vi "参数配置表.vi"() -> ()   [LabVIEW 2016, in "数据传输系统-05.lvlib"]
uses:
  <vilib>/Utility/miscctls.llb/LVPointTypeDef.ctl
  <vilib>/ptbypt/NI_PtbyPt.lvlib
panel:
  in  "加密传输":bool
  in  "数据库类型":enum16{"Access", "SQLite"}(ring)
  in  "应用环境":enum16{"STD", "GB212"}(ring)
  in  "屏蔽维护数据":bool
  in  "数据发送延时时间/s":i32
  in  "判断数据反馈":enum16{"非严格判断", "严格判断", "不判断"}(ring)
  in  "仪器参数发送":bool
  in  "地表水/污染源":bool
  in  "间隔时间/分钟":i32
  in  "数据发送通道":enum16{"TCP", "VISA"}(ring)
  in  "数据发送协议":enum16{"2005-212协议", "2017-212协议"}(ring)=enum."2017-212协议"
  in  "数据触发上传方式":enum16{"出数即刻发送", "间隔时间发送", "整点发送"}(ring)
  in  "数据组合发送":bool
  in  "日志、参数发送":bool
  in  "2011发送":bool
  in  "返回":bool
  out "配置表格":string[][](table)
  in  "参数数值":T1={"CODMn"=TRUE, "CODCr"=TRUE, "DO"=TRUE, "铜"=TRUE, "PH"=TRUE, "氨氮"=TRUE, "比电导率"=TRUE, "水温"=TRUE, "COD"=TRUE, "浊度"=TRUE, "总氮"=TRUE, "总磷"=TRUE, "叶绿素a"=TRUE, "藻密度"=TRUE, "水位"=TRUE, "流速"=TRUE, "瞬时流量"=TRUE, "累积流量"=TRUE, "亚硝氮"=TRUE, "硫化物"=TRUE, "ORP"=TRUE, "铅"=TRUE, "镉"=TRUE, "锌"=TRUE, "镍"=TRUE, "锰"=TRUE, "汞"=TRUE, "气温"=TRUE, "气压"=TRUE, "风速"=TRUE, "风向"=TRUE, "盐度"=TRUE, "磷酸盐"=TRUE, "硝氮"=TRUE, "氟化物"=TRUE}
  # "因子编码，单位配置，上传功能码，小时、质控数据上传触发方式"
  # "参数配置"
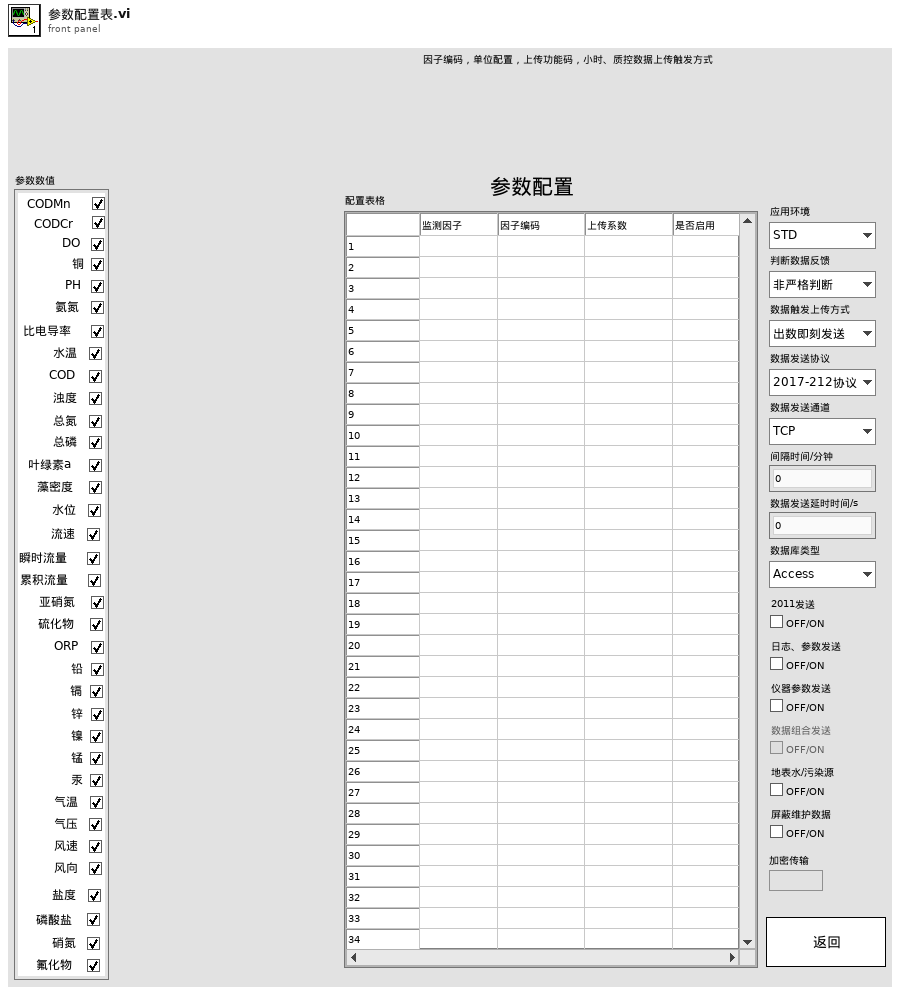
[diagram p1: front panel]
types:
  T1 = cluster{"CODMn":bool, "CODCr":bool, "DO":bool, "铜":bool, "PH":bool, "氨氮":bool, "比电导率":bool, "水温":bool, "COD":bool, "浊度":bool, "总氮":bool, "总磷":bool, "叶绿素a":bool, "藻密度":bool, "水位":bool, "流速":bool, "瞬时流量":bool, "累积流量":bool, "亚硝氮":bool, "硫化物":bool, "ORP":bool, "铅":bool, "镉":bool, "锌":bool, "镍":bool, "锰":bool, "汞":bool, "气温":bool, "气压":bool, "风速":bool, "风向":bool, "盐度":bool, "磷酸盐":bool, "硝氮":bool, "氟化物":bool}
  T2 = typedef "LVPointTypeDef.ctl" = cluster{"Horizontal":i16, "Vertical":i16}
  T3 = cluster{"[0]":string, "[1]":string, "[2]":string, "[3]":string, "[4]":string, "[5]":string, "[6]":string, "[7]":string, "[8]":string, "[9]":string, "[10]":string, "[11]":string, "[12]":string, "[13]":string, "[14]":string, "[15]":string, "[16]":string, "[17]":string, "[18]":string, "[19]":string, "[20]":string, "[21]":string, "[22]":string, "[23]":string, "[24]":string, "[25]":string, "[26]":string, "[27]":string, "[28]":string, "[29]":string, "[30]":string, "[31]":string, "[32]":string, "[33]":string, "[34]":string}
  T4 = enum8{"Enabled", "Disabled", "Disabled and Grayed Out"}
  T5 = typedef "LVRowAndColumnTypeDef.ctl" = cluster{"Row":i32, "Column":i32}
  T6 = cluster{"[0]":string, "[1]":string, "[2]":string, "[3]":string, "[4]":string, "[5]":string, "[6]":string}
  T7 = cluster{"[0]":string, "[1]":string, "[2]":string, "[3]":string, "[4]":string, "[5]":string, "[6]":string, "[7]":string, "[8]":string, "[9]":string, "[10]":string, "[11]":string, "[12]":string}
  T8 = cluster{"[0]":string, "[1]":string, "[2]":string, "[3]":string, "[4]":string, "[5]":string, "[6]":string, "[7]":string, "[8]":string, "[9]":string, "[10]":string, "[11]":string, "[12]":string, "[13]":string}
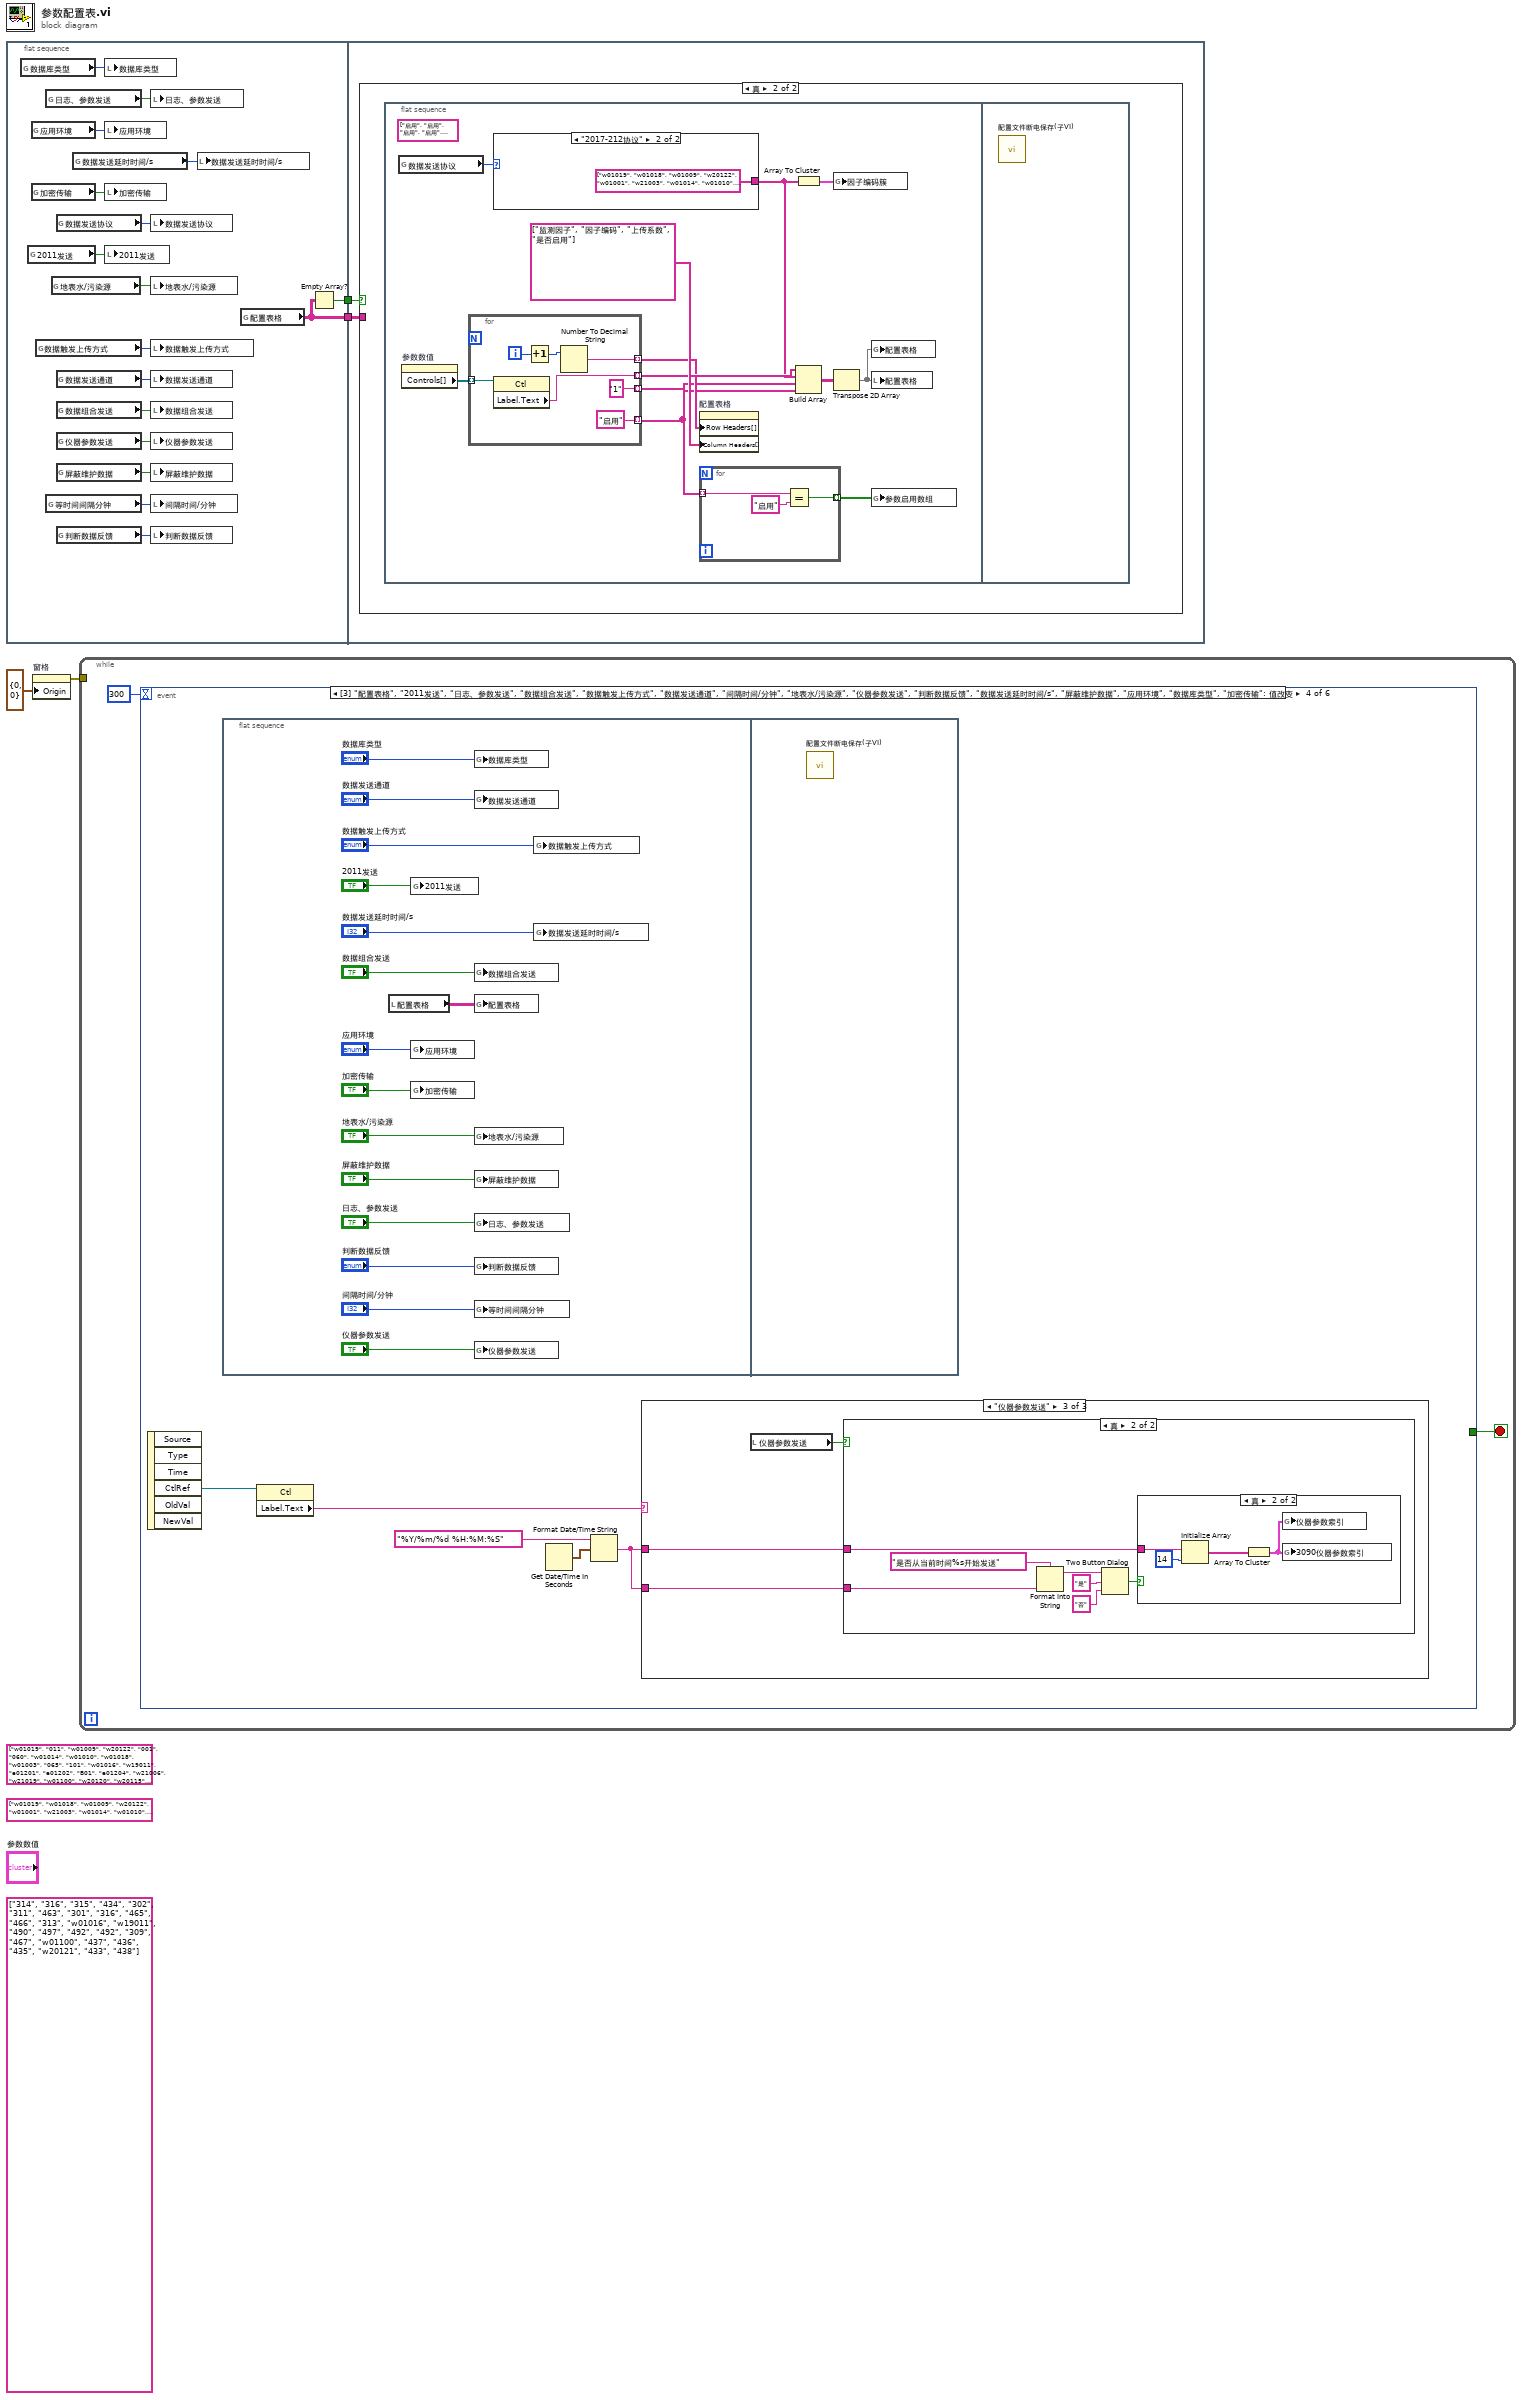
[diagram p0: block diagram]
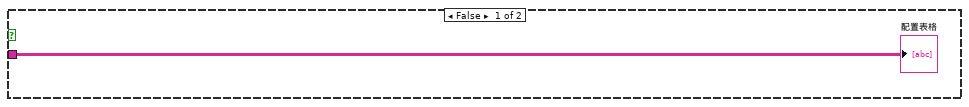
[diagram p2: hidden frame]
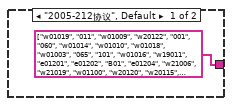
[diagram p3: hidden frame]
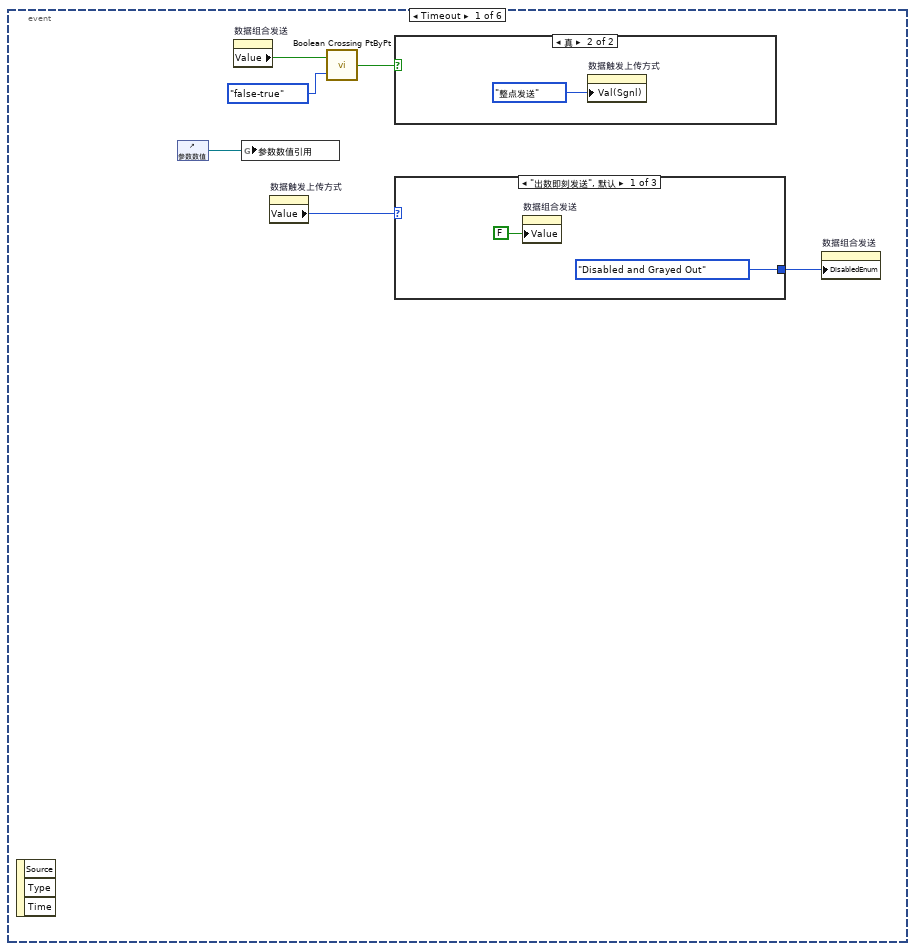
[diagram p4: hidden frame]
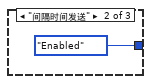
[diagram p6: hidden frame]
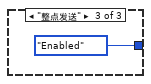
[diagram p7: hidden frame]
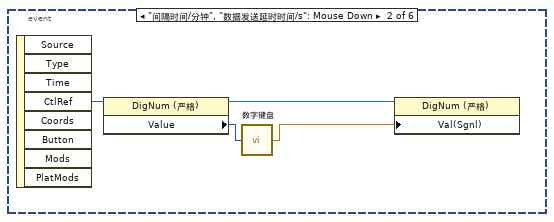
[diagram p8: hidden frame]
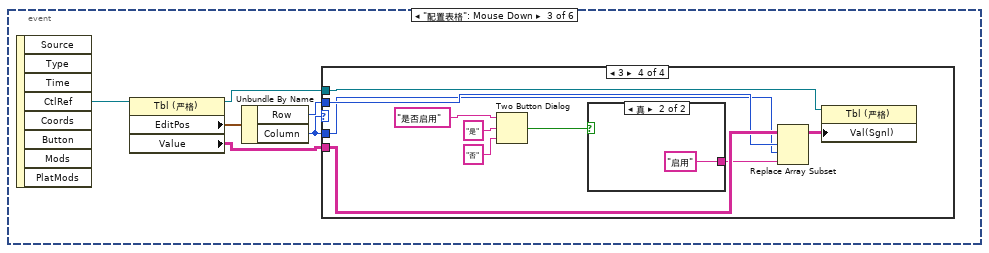
[diagram p9: hidden frame]
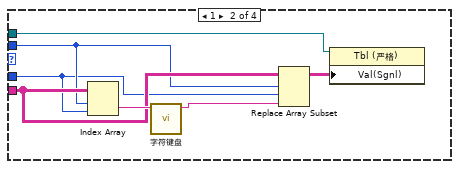
[diagram p11: hidden frame]
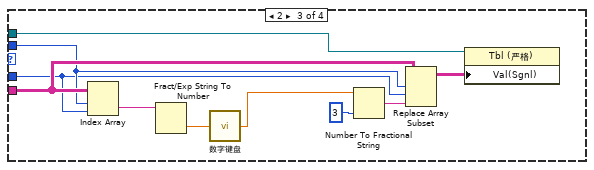
[diagram p12: hidden frame]
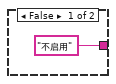
[diagram p13: hidden frame]
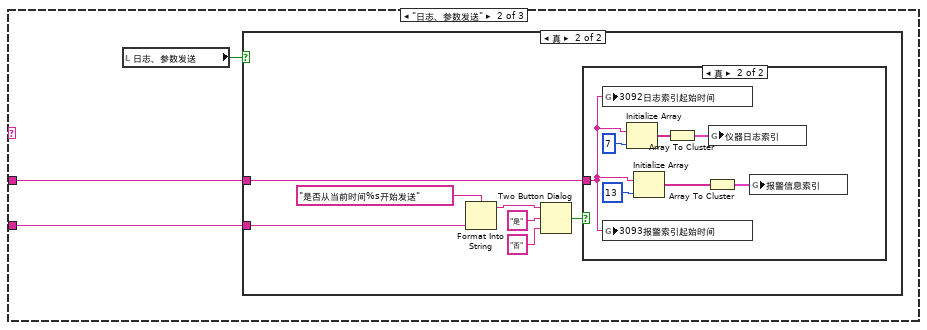
[diagram p15: hidden frame]
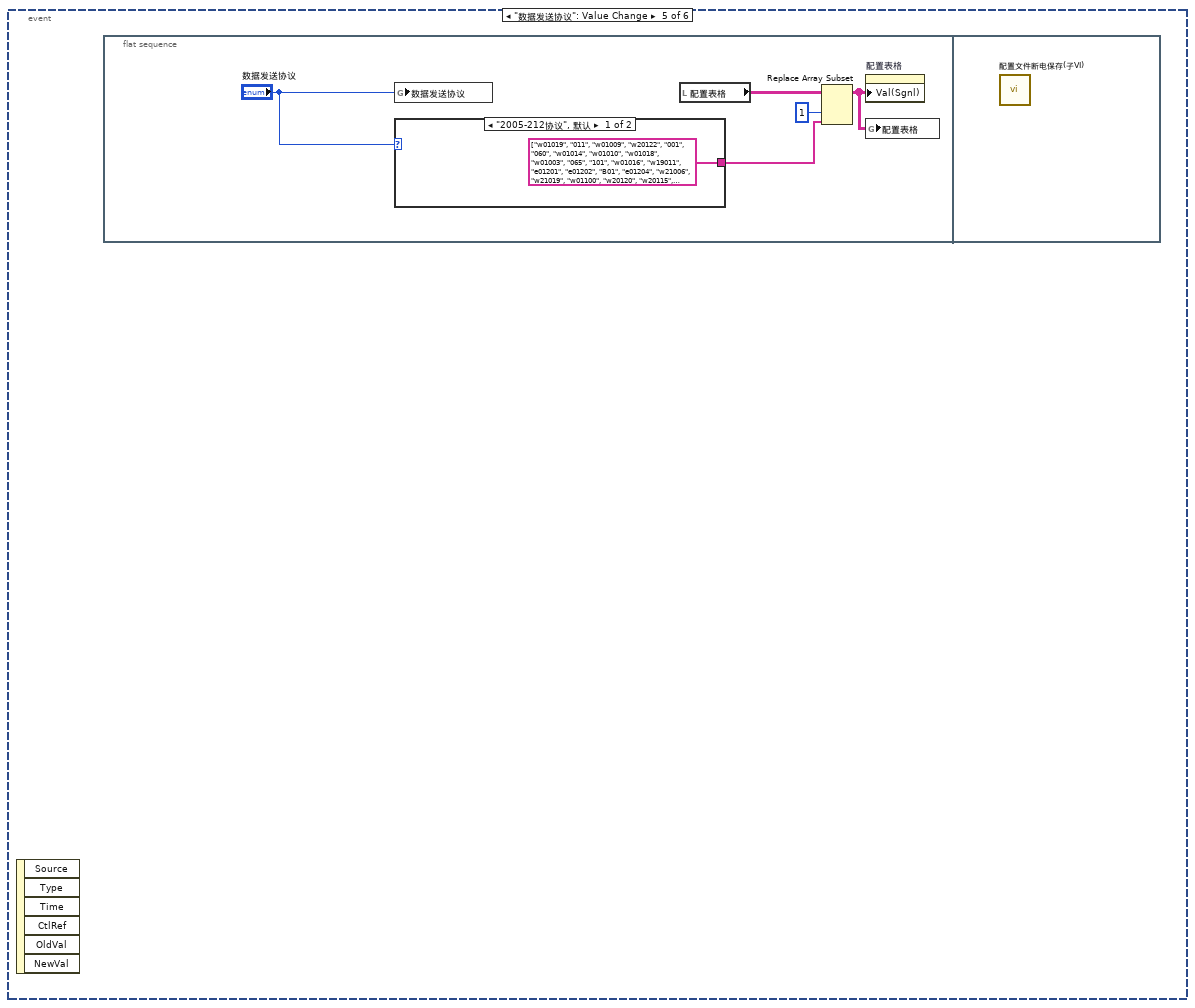
[diagram p20: hidden frame]
diagram:
  (unwired) string[] ["w01019", "011", "w01009", "w20122", "001", "060", "w01014", "w01010", "w01018", "w01003", "065", "101", "w01016", "w19011", "e01201", "e01202", "B01", "e01204", "w21006", "w21019", "w01100", "w20120", "w20115", "w20123", "w20121", "w20124", "w20111", "a01001", "a01006", "a01007", "a01008", "w01002", "w21015", "w21007", "w21017"]
  (unwired) string[] ["w01019", "w01018", "w01009", "w20122", "w01001", "w21003", "w01014", "w01010", "w01018", "w01003", "w21001", "w21011", "w01016", "w19011", "e01201", "e01202", "e01203", "e01204", "w21006", "w21019", "w01100", "w20120", "w20115", "w20123", "w20121", "w20124", "w20111", "a01001", "a01006", "a01007", "a01008", "w01002", "w21015", "w21007", "w21017"]
  (unwired) string[] ["314", "316", "315", "434", "302", "311", "463", "301", "316", "465", "466", "313", "w01016", "w19011", "490", "497", "492", "492", "309", "467", "w01100", "437", "436", "435", "w20121", "433", "438"]
  n1 = flat-sequence {
    tunnel: [w14] -> w2
    tunnel: [w13] -> w1
    tunnel: w2 -> [w23]
    tunnel: w1 -> [w22]
    frame #0 {
      n2 = global read "断电保存全局.vi" "数据库类型"() -> (w6:enum16{"Access", "SQLite"})
      n3 = global read "断电保存全局.vi" "2011发送"() -> (w21:bool)
      n4 = global read "断电保存全局.vi" "应用环境"() -> (w7:enum16{"STD", "GB212"})
      n5 = global read "断电保存全局.vi" "加密传输"() -> (w5:bool)
      n6 = global read "断电保存全局.vi" "数据触发上传方式"() -> (w17:enum16{"出数即刻发送", "间隔时间发送", "整点发送"})
      n7 = global read "断电保存全局.vi" "日志、参数发送"() -> (w19:bool)
      n8 = global read "断电保存全局.vi" "等时间间隔分钟"() -> (w12:i32)
      n9 = global read "断电保存全局.vi" "地表水/污染源"() -> (w11:bool)
      n10 = global read "断电保存全局.vi" "数据发送协议"() -> (w15:enum16{"2005-212协议", "2017-212协议"})
      n11 = global read "断电保存全局.vi" "数据发送通道"() -> (w16:enum16{"TCP", "VISA"})
      n12 = global read "断电保存全局.vi" "数据组合发送"() -> (w18:bool)
      n13 = global read "断电保存全局.vi" "仪器参数发送"() -> (w10:bool)
      n14 = global read "断电保存全局.vi" "屏蔽维护数据"() -> (w8:bool)
      n15 = global read "断电保存全局.vi" "判断数据反馈"() -> (w20:enum16{"非严格判断", "严格判断", "不判断"})
      n16 = global read "断电保存全局.vi" "数据发送延时时间/s"() -> (w9:i32)
      n17 = local write "数据库类型"(w6) -> ()
      n18 = local write "应用环境"(w7) -> ()
      n19 = local write "加密传输"(w5) -> ()
      n20 = local write "2011发送"(w21) -> ()
      n21 = local write "日志、参数发送"(w19) -> ()
      n22 = local write "数据发送协议"(w15) -> ()
      n23 = local write "地表水/污染源"(w11) -> ()
      n24 = local write "数据触发上传方式"(w17) -> ()
      n25 = local write "数据发送通道"(w16) -> ()
      n26 = local write "数据组合发送"(w18) -> ()
      n27 = local write "仪器参数发送"(w10) -> ()
      n28 = local write "屏蔽维护数据"(w8) -> ()
      n29 = local write "间隔时间/分钟"(w12) -> ()
      n30 = local write "判断数据反馈"(w20) -> ()
      n31 = local write "数据发送延时时间/s"(w9) -> ()
      n32 = global read "断电保存全局.vi" "配置表格"() -> (w13:string[][])
      n33 = Empty Array?(array=w13) -> (empty?=w14:bool)
    }
    frame #1 {
      n34 = case shown="真" w23 {
        tunnel: w22 -> [w24 _]
        frame False {
          "配置表格" <- w24
        }
        frame True {
          n35 = flat-sequence {
            frame #0 {
              (unwired) string[] ["启用", "启用", "启用", "启用", "启用", "启用", "启用", "启用", "启用", "启用", "启用", "启用", "启用", "启用", "启用", "启用", "启用", "启用", "启用", "启用", "启用", "启用", "启用", "启用", "启用", "启用", "启用"]
              n36 = global read "断电保存全局.vi" "数据发送协议"() -> (w30:enum16{"2005-212协议", "2017-212协议"})
              n37 = property on="参数数值" class="Clust (严格)"() -> ("Controls[]"=w32:refnum<vi>[])  [unwired: 2 in, 2 out]
              n38 = for {
                tunnel: w32 -> [w48] mode=indexing
                tunnel: [w47] -> w34 mode=indexing
                tunnel: [w45] -> w33 mode=indexing
                tunnel: ["1"] -> w27 mode=indexing
                tunnel: ["启用"] -> w25 mode=indexing
                i -> [w46]
                n39 = property class="Ctl"(reference=w48) -> ("Label.Text"=w47:string)  [unwired: 1 in, 2 out]
                n40 = Increment(x=w46) -> (x+1=w44:i32)
                n41 = Number To Decimal String(number=w44) -> (decimal integer string=w45:string)  [unwired: 1 in]
              }
              n42 = case shown="\"2017-212协议\"" w30 {
                tunnel: [string[] ["w01019", "011", "w01009", "w20122", "001", "060", "w01014", "w01010", "w01018", "w01003", "065", "101", "w01016", "w19011", "e01201", "e01202", "B01", "e01204", "w21006", "w21019", "w01100", "w20120", "w20115", "w20123", "w20121", "w20124", "w20111", "a01001", "a01006", "a01007", "a01008", "w01002", "w21015", "w21007", "w21017"] string[] ["w01019", "w01018", "w01009", "w20122", "w01001", "w21003", "w01014", "w01010", "w01018", "w01003", "w21001", "w21011", "w01016", "w19011", "e01201", "e01202", "e01203", "e01204", "w21006", "w21019", "w01100", "w20120", "w20115", "w20123", "w20121", "w20124", "w20111", "a01001", "a01006", "a01007", "a01008", "w01002", "w21015", "w21007", "w21017"]] -> w28
                frame "2005-212协议", Default {
                }
                frame "2017-212协议" {
                }
              }
              n43 = property on="配置表格" class="Tbl (严格)"("Row Headers[]"=w33, "Column Headers[]"=string[] ["监测因子", "因子编码", "上传系数", "是否启用"]) -> ()  [unwired: 2 in, 2 out]
              n44 = for {
                tunnel: w25 -> [w39] mode=indexing
                tunnel: [w37] -> w26 mode=indexing
                n45 = Equal?(x=w39, y="启用") -> (x = y?=w37:bool)
              }
              n46 = Array To Cluster(array=w28) -> (cluster=w29:T3)
              n47 = Build Array(w34, w28, w27, w25) -> (w36:string[][])
              n48 = global write "断电保存全局.vi" "因子编码簇"(w29) -> ()
              n49 = Transpose 2D Array(2D array=w36) -> (transposed array=w31:string[][])
              n50 = global write "断电保存全局.vi" "配置表格"(w31) -> ()
              n51 = local write "配置表格"(w31) -> ()
              n52 = global write "断电保存全局.vi" "参数启用数组"(w26) -> ()
            }
            frame #1 {
              n53 = call "配置文件断电保存(子VI).vi"() -> ()  [unwired: 12 in]
            }
          }
        }
      }
    }
  }
  n54 = property on="窗格" class="Pane"("Origin"=T2 {"Horizontal"=0, "Vertical"=0} ("原点")) -> (error out=w4:errorcluster)  [unwired: 2 in, 1 out]
  n55 = while {
    tunnel: w4 -> [_]
    stop <- w49 stop-if-true
    n56 = event shown="[3] \"配置表格\", \"2011发送\", \"日志、参数发送\", \"数据组合发送\", \"数据触发上传方式\", \"数据发送通道\", \"间隔时间/分钟\", \"地表水/污染源\", \"仪器参数发送\", \"判断数据反馈\", \"数据发送延时时间/s\", \"屏蔽维护数据\", \"应用环境\", \"数据库类型\", \"加密传输\": 值改变" {
      selector: _ -> [_ _ _ _ _ _]
      dyn-events: _ -> [_ _ _ _ _ _]
      timeout: 300 -> [_ _ _ _ _ _]
      tunnel: [_ _ _ _ _ TRUE] -> w49
      event Timeout {
        n57 = event-data() -> ()  [unwired: 1 in, 3 out]
        n58 = control-ref of="参数数值"() -> (w51:refnum<vi>)
        n59 = property on="数据组合发送" class="Bool (严格)"() -> ("Value"=w54:bool)  [unwired: 2 in, 2 out]
        n60 = global write "断电保存全局.vi" "参数数值引用"(w51) -> ()
        n61 = property on="数据触发上传方式" class="Enum (严格)"() -> ("Value"=w56:enum16{"出数即刻发送", "间隔时间发送", "整点发送"})  [unwired: 2 in, 2 out]
        n62 = call <vilib>:"Boolean Crossing PtByPt.vi"("direction"=enum16{"either", "false-true", "true-false"}."false-true", "input"=w54) -> ("crossing"=w52:bool)  [unwired: 1 in]
        n63 = case shown="真" w52 {
          frame False {
          }
          frame True {
            n64 = property on="数据触发上传方式" class="Enum (严格)"("Val(Sgnl)"=enum16{"出数即刻发送", "间隔时间发送", "整点发送"}."整点发送" ("值(信号)")) -> ()  [unwired: 2 in, 2 out]
          }
        }
        n65 = case shown="\"出数即刻发送\", 默认" w56 {
          tunnel: [T4."Disabled and Grayed Out" ("禁用") T4."Enabled" ("禁用") T4."Enabled" ("禁用")] -> w55
          frame "出数即刻发送", Default {
            n66 = property on="数据组合发送" class="Bool (严格)"("Value"=FALSE ("值(信号)")) -> ()  [unwired: 2 in, 2 out]
          }
          frame "间隔时间发送" {
          }
          frame "整点发送" {
          }
        }
        n67 = property on="数据组合发送" class="Bool (严格)"("DisabledEnum"=w55) -> ()  [unwired: 2 in, 2 out]
      }
      event "间隔时间/分钟", "数据发送延时时间/s": Mouse Down {
        n68 = event-data() -> ("CtlRef"=w65:refnum<vi>)  [unwired: 1 in, 7 out]
        n69 = property class="DigNum (严格)"(reference=w65) -> (reference out=w63:refnum<vi>, "Value"=w64:i32)  [unwired: 1 in, 1 out]
        n70 = call "数字键盘.vi"("OldNumber"=w64) -> ("NewNumber"=w62:sgl)
        n71 = property class="DigNum (严格)"(reference=w63, "Val(Sgnl)"=w62) -> ()  [unwired: 1 in, 2 out]
      }
      event "配置表格": Mouse Down {
        n72 = event-data() -> ("CtlRef"=w71:refnum<vi>)  [unwired: 1 in, 7 out]
        n73 = property class="Tbl (严格)"(reference=w71) -> (reference out=w67:refnum<vi>, "EditPos"=w70:T5, "Value"=w69:string[][])  [unwired: 1 in, 1 out]
        n74 = Unbundle By Name(w70) -> ("Row"=w68:i32, "Column"=w66:i32)
        n75 = case shown="3" w66 {
          tunnel: w69 -> [_ w77 w88 w92]
          tunnel: w68 -> [_ w76 w87 w91]
          tunnel: w66 -> [_ w75 w86 w90]
          tunnel: w67 -> [_ w73 w85 w93]
          frame 0, Default {
          }
          frame 1 {
            n76 = Index Array(array=w77, index (row)=w76, index (col)=w75) -> (element=w78:string)
            n77 = call "字符键盘.vi"("原值"=w78) -> ("x+y"=w74:string)  [unwired: 10 in]
            n78 = Replace Array Subset(array=w77, new element=w74, index (row)=w76, index (col)=w75) -> (w72:string[][])
            n79 = property class="Tbl (严格)"(reference=w73, "Val(Sgnl)"=w72) -> ()  [unwired: 1 in, 2 out]
          }
          frame 2 {
            n80 = Index Array(array=w88, index (row)=w87, index (col)=w86) -> (element=w83:string)
            n81 = Fract/Exp String To Number(string=w83) -> (number=w82:dbl)  [unwired: 3 in, 1 out]
            n82 = call "数字键盘.vi"("OldNumber"=w82) -> ("NewNumber"=w81:sgl)
            n83 = Number To Fractional String(number=w81, precision (6)=i16 3 ("精度(6)")) -> (F-format string=w80:string)  [unwired: 2 in]
            n84 = Replace Array Subset(array=w88, new element=w80, index (row)=w87, index (col)=w86) -> (w84:string[][])
            n85 = property class="Tbl (严格)"(reference=w85, "Val(Sgnl)"=w84) -> ()  [unwired: 1 in, 2 out]
          }
          frame 3 {
            n86 = Two Button Dialog(message="是否启用" ("消息"), 1:"否" ("F按钮名称（“取消”）"), 2:"是" ("T按钮名称（“确定”）")) -> (T button?=w95:bool)
            n87 = case shown="真" w95 {
              tunnel: ["不启用" "启用"] -> w89
              frame False {
              }
              frame True {
              }
            }
            n88 = Replace Array Subset(array=w92, new element=w89, index (row)=w91, index (col)=w90) -> (w94:string[][])
            n89 = property class="Tbl (严格)"(reference=w93, "Val(Sgnl)"=w94) -> ()  [unwired: 1 in, 2 out]
          }
        }
      }
      event "配置表格", "2011发送", "日志、参数发送", "数据组合发送", "数据触发上传方式", "数据发送通道", "间隔时间/分钟", "地表水/污染源", "仪器参数发送", "判断数据反馈", "数据发送延时时间/s", "屏蔽维护数据", "应用环境", "数据库类型", "加密传输": Value Change {
        n90 = event-data() -> ("CtlRef"=w105:refnum<vi>)  [unwired: 1 in, 5 out]
        n91 = flat-sequence {
          frame #0 {
            n92 = local read "配置表格"() -> (w151:string[][])
            n93 = global write "断电保存全局.vi" "2011发送"("2011发送") -> ()
            n94 = global write "断电保存全局.vi" "应用环境"("应用环境") -> ()
            n95 = global write "断电保存全局.vi" "加密传输"("加密传输") -> ()
            n96 = global write "断电保存全局.vi" "数据库类型"("数据库类型") -> ()
            n97 = global write "断电保存全局.vi" "数据发送通道"("数据发送通道") -> ()
            n98 = global write "断电保存全局.vi" "数据组合发送"("数据组合发送") -> ()
            n99 = global write "断电保存全局.vi" "配置表格"(w151) -> ()
            n100 = global write "断电保存全局.vi" "地表水/污染源"("地表水/污染源") -> ()
            n101 = global write "断电保存全局.vi" "屏蔽维护数据"("屏蔽维护数据") -> ()
            n102 = global write "断电保存全局.vi" "日志、参数发送"("日志、参数发送") -> ()
            n103 = global write "断电保存全局.vi" "判断数据反馈"("判断数据反馈") -> ()
            n104 = global write "断电保存全局.vi" "等时间间隔分钟"("间隔时间/分钟") -> ()
            n105 = global write "断电保存全局.vi" "仪器参数发送"("仪器参数发送") -> ()
            n106 = global write "断电保存全局.vi" "数据触发上传方式"("数据触发上传方式") -> ()
            n107 = global write "断电保存全局.vi" "数据发送延时时间/s"("数据发送延时时间/s") -> ()
          }
          frame #1 {
            n108 = call "配置文件断电保存(子VI).vi"() -> ()  [unwired: 12 in]
          }
        }
        n109 = property class="Ctl"(reference=w105) -> ("Label.Text"=w104:string)  [unwired: 1 in, 2 out]
        n110 = Get Date/Time In Seconds() -> (seconds since 1Jan1904=w103:timestamp)
        n111 = Format Date/Time String(time format string (%c)="%Y/%m/%d %H:%M:%S" ("时间格式字符串(%c)"), seconds (now)=w103) -> (date/time string=w101:string)  [unwired: 1 in]
        n112 = case shown="\"仪器参数发送\"" w104 {
          tunnel: w101 -> [_ w107 w124]
          tunnel: w101 -> [_ w106 w123]
          frame "假", Default {
          }
          frame "日志、参数发送" {
            n113 = local read "日志、参数发送"() -> (w108:bool)
            n114 = case shown="真" w108 {
              tunnel: w107 -> [_ w112]
              tunnel: w106 -> [_ w110]
              frame False {
              }
              frame True {
                n115 = Format Into String(format string="是否从当前时间%s开始发送" ("消息"), w110) -> (resulting string=w109:string)  [unwired: 2 in, 1 out]
                n116 = Two Button Dialog(message=w109, 1:"否" ("F按钮名称（“取消”）"), 2:"是" ("T按钮名称（“确定”）")) -> (T button?=w113:bool)
                n117 = case shown="真" w113 {
                  tunnel: w112 -> [_ w116]
                  frame False {
                  }
                  frame True {
                    n118 = global write "全局 时间2.vi" "3092日志索引起始时间"(w116) -> ()
                    n119 = global write "全局 时间2.vi" "3093报警索引起始时间"(w116) -> ()
                    n120 = Initialize Array(w116, 7 ("维数大小")) -> (w117:string[])
                    n121 = Initialize Array(w116, 13 ("维数大小")) -> (w120:string[])
                    n122 = Array To Cluster(array=w117) -> (cluster=w118:T6)
                    n123 = Array To Cluster(array=w120) -> (cluster=w119:T7)
                    n124 = global write "全局 时间2.vi" "仪器日志索引"(w118) -> ()
                    n125 = global write "全局 时间2.vi" "报警信息索引"(w119) -> ()
                  }
                }
              }
            }
          }
          frame "仪器参数发送" {
            n126 = local read "仪器参数发送"() -> (w125:bool)
            n127 = case shown="真" w125 {
              tunnel: w124 -> [_ w129]
              tunnel: w123 -> [_ w127]
              frame False {
              }
              frame True {
                n128 = Format Into String(format string="是否从当前时间%s开始发送" ("消息"), w127) -> (resulting string=w126:string)  [unwired: 2 in, 1 out]
                n129 = Two Button Dialog(message=w126, 1:"否" ("F按钮名称（“取消”）"), 2:"是" ("T按钮名称（“确定”）")) -> (T button?=w130:bool)
                n130 = case shown="真" w130 {
                  tunnel: w129 -> [_ w134]
                  frame False {
                  }
                  frame True {
                    n131 = Initialize Array(w134, 14 ("维数大小")) -> (w136:string[])
                    n132 = Array To Cluster(array=w136) -> (cluster=w133:T8)
                    n133 = global write "全局 时间2.vi" "仪器参数索引"(w133) -> ()
                    n134 = global write "全局 时间2.vi" "3090仪器参数索引"(w133) -> ()
                  }
                }
              }
            }
          }
        }
      }
      event "数据发送协议": Value Change {
        n135 = event-data() -> ()  [unwired: 1 in, 6 out]
        n136 = flat-sequence {
          frame #0 {
            n137 = global write "断电保存全局.vi" "数据发送协议"("数据发送协议") -> ()
            n138 = case shown="\"2005-212协议\", 默认" "数据发送协议" {
              tunnel: [string[] ["w01019", "011", "w01009", "w20122", "001", "060", "w01014", "w01010", "w01018", "w01003", "065", "101", "w01016", "w19011", "e01201", "e01202", "B01", "e01204", "w21006", "w21019", "w01100", "w20120", "w20115", "w20123", "w20121", "w20124", "w20111", "a01001", "a01006", "a01007", "a01008", "w01002", "w21015", "w21007", "w21017"] string[] ["w01019", "w01018", "w01009", "w20122", "w01001", "w21003", "w01014", "w01010", "w01018", "w01003", "w21001", "w21011", "w01016", "w19011", "e01201", "e01202", "e01203", "e01204", "w21006", "w21019", "w01100", "w20120", "w20115", "w20123", "w20121", "w20124", "w20111", "a01001", "a01006", "a01007", "a01008", "w01002", "w21015", "w21007", "w21017"]] -> w154
              frame "2005-212协议", Default {
              }
              frame "2017-212协议" {
              }
            }
            n139 = local read "配置表格"() -> (w155:string[][])
            n140 = Replace Array Subset(array=w155, new element=w154, index (col)=1 ("禁用的索引 (列)")) -> (w152:string[][])  [unwired: 1 in]
            n141 = property on="配置表格" class="Tbl (严格)"("Val(Sgnl)"=w152) -> ()  [unwired: 2 in, 2 out]
            n142 = global write "断电保存全局.vi" "配置表格"(w152) -> ()
          }
          frame #1 {
            n143 = call "配置文件断电保存(子VI).vi"() -> ()  [unwired: 12 in]
          }
        }
      }
      event "返回": Value Change; Panel Close {
        n144 = event-data() -> ()  [unwired: 1 in, 3 out]
      }
    }
  }
